vi "vision logic.vi"() -> ()   [LabVIEW 2018]
uses:
  <vilib>/Rock Robotics/Network Tables/NT Read Number.vi
  <vilib>/Rock Robotics/Network Tables/NT Read Boolean.vi
  <vilib>/Rock Robotics/Network Tables/NT Write Number.vi
  <vilib>/Rock Robotics/Network Tables/NT Write Boolean.vi
  <vilib>/Rock Robotics/WPI/Utilities/WPI_GetSetVariantRefNum.vi
  <vilib>/Rock Robotics/Network Tables/NT Write Numeric Array.vi
panel:
  out "RobotDrive Motors":dbl
  in  "Tab Control":T1(tab)
  in  "High Threshold":dbl=0.68
  in  "Low Threshold":dbl=0.63
  out "Center of Centroid":dbl
  out "Sonar1 Value":dbl
  in  "Wall (Sonar)":dbl=3.0
  in  "LX axis":dbl=0.6000000000000001 min=-1.0 max=1.0 step=0.05
  in  "LY axis":dbl=-0.45 min=-1.0 max=1.0 step=0.05
  in  "RX axis":dbl=0.45 min=-1.0 max=1.0 step=0.05
  in  "RY axis":dbl=-0.6000000000000001 min=-1.0 max=1.0 step=0.05
  in  "X axis":dbl=0.45 min=-1.0 max=1.0 step=0.05
  in  "Y axis":dbl=-0.45 min=-1.0 max=1.0 step=0.05
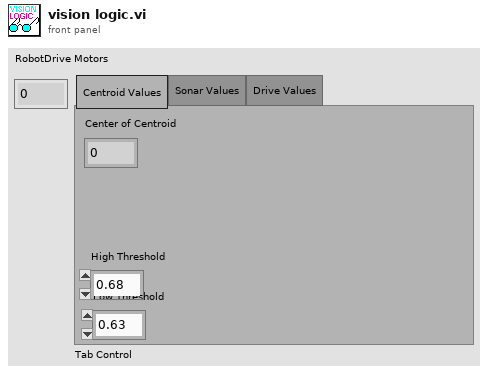
[diagram p1: front panel]
types:
  T1 = enum32{"Centroid Values", "Sonar Values", "Drive Values"}
  T2 = typedef "WPI_RobotDriveDevRef.ctl" = cluster{"DevStatus":errorcluster, "Motors[]":T3[], "Square Inputs":bool, "Max Output":dbl}
  T3 = typedef "WPI_MotorControlDeviceRef.ctl" = cluster{"DeviceStatus":errorcluster, "Type":T4, "PWM":cluster{"PWM Channel":T5, "DeadBand":T6}, "CAN":cluster{"Device Number":u8, "SetOutput VI Ref":variant, "GetOutput VI Ref":variant, "Enable VI Ref":variant, "Disable VI Ref":variant, "Data":variant}, "Invert":bool, "DIO PWM":cluster{"PWM \"Enable\" Channel":T5, "DIOChannel":T7, "PWM Rate":dbl}}
  T4 = typedef "WPI_MotorControlType.ctl" = enum16{"PWM", "CAN", "DIO PWM"}
  T5 = typedef "FPGA_DIOPWMChannel.ctl" = enum8{"PWM 0", "PWM 1", "PWM 2", "PWM 3", "PWM 4", "PWM 5", "PWM 6", "PWM 7", "PWM 8", "PWM 9", "PWM MXP 0", "PWM MXP 1", "PWM MXP 2", "PWM MXP 3", "PWM MXP 4", "PWM MXP 5", "PWM MXP 6", "PWM MXP 7", "PWM MXP 8", "PWM MXP 9", "Invalid"}
  T6 = typedef "WPI_PWMDeadband.ctl" = cluster{"Name":string, "maxPositivePwm":i32, "minPositivePwm":i32, "centerPwm":i32, "maxNegativePwm":i32, "minNegativePwm":i32, "angularRange":u16}
  T7 = typedef "FPGA_DIOChannel.ctl" = enum8{"DIO 0", "DIO 1", "DIO 2", "DIO 3", "DIO 4", "DIO 5", "DIO 6", "DIO 7", "DIO 8", "DIO 9", "DIO MXP 0", "DIO MXP 1", "DIO MXP 2", "DIO MXP 3", "DIO MXP 4", "DIO MXP 5", "DIO MXP 6", "DIO MXP 7", "DIO MXP 8", "DIO MXP 9", "DIO MXP 10", "DIO MXP 11", "DIO MXP 12", "DIO MXP 13", "DIO MXP 14", "DIO MXP 15", "SPI Port CS1", "SPI Port CS2", "SPI Port CS3", "SPI Port MISO", "SPI Port MOSI", "Invalid"}
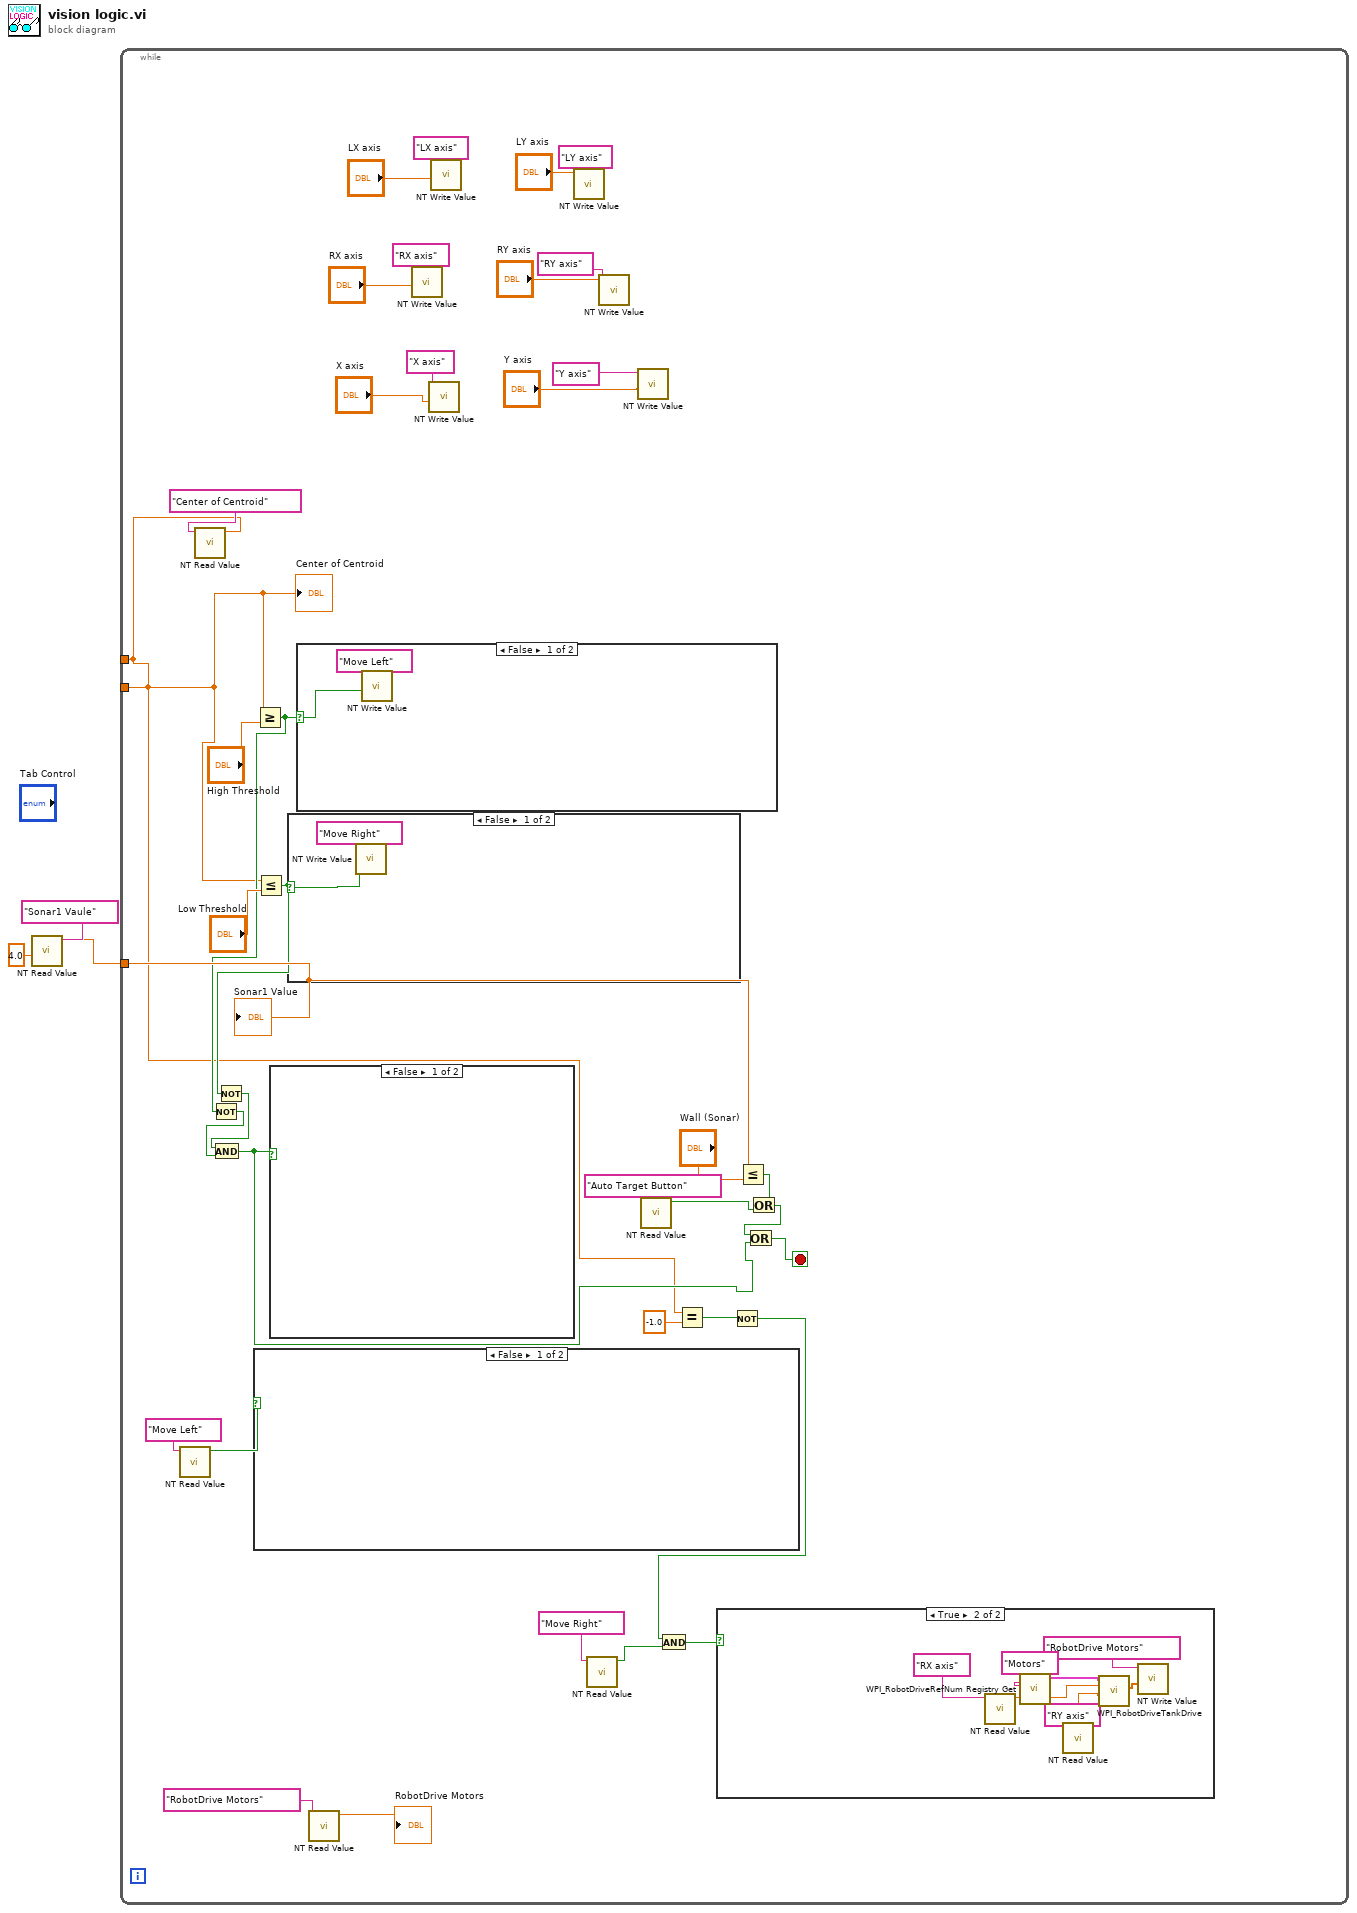
[diagram p0: block diagram]
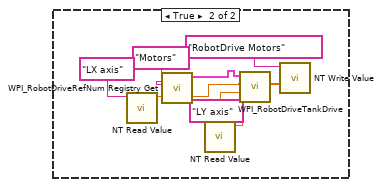
[diagram p3: hidden frame]
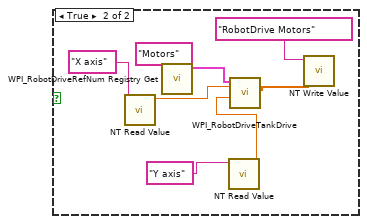
[diagram p4: hidden frame]
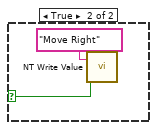
[diagram p5: hidden frame]
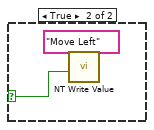
[diagram p6: hidden frame]
diagram:
  n1 = call-poly <vilib>:"NT Read Value.vi"("Default Value"=4.0, "Name"="Sonar1 Vaule") -> ("Numeric"=w2:dbl)  [unwired: 8 in, 1 out]
  n2 = while {
    tunnel: w2 -> [w36]
    tunnel: [w4] -> _
    tunnel: [w4] -> _
    stop <- w12 stop-if-true
    n3 = call-poly <vilib>:"NT Read Value.vi"("Name"="Move Left") -> ("Boolean"=w30:bool)  [unwired: 9 in, 1 out]
    n4 = call-poly <vilib>:"NT Read Value.vi"("Name"="Center of Centroid") -> ("Numeric"=w4:dbl)  [unwired: 9 in, 1 out]
    "Center of Centroid" <- w4
    n5 = case shown="False" w30 {
      frame False {
      }
      frame True {
        n6 = call-poly <vilib>:"NT Read Value.vi"("Name"="LX axis") -> ("Numeric"=w51:dbl)  [unwired: 9 in, 1 out]
        n7 = call <vilib>:"WPI_RobotDriveRefNum Registry Get.vi"("refnum name"="Motors") -> ("RobotDriveDevRef"=w52:T2)  [unwired: 1 in, 9 out]
        n8 = call-poly <vilib>:"NT Read Value.vi"("Name"="LY axis") -> ("Numeric"=w50:dbl)  [unwired: 9 in, 1 out]
        n9 = call <vilib>:"WPI_RobotDriveTankDrive.vi"("Right axis value"=w50, "Left axis value"=w51, "RobotDriveDevRef"=w52) -> ("Motor Values"=w53:dbl[])  [unwired: 6 in, 2 out]
        n10 = call-poly <vilib>:"NT Write Value.vi"("Numeric Array"=w53, "Name"="RobotDrive Motors") -> ()  [unwired: 9 in, 1 out]
      }
    }
    n11 = Greater Or Equal?(x=w4, y="High Threshold") -> (x >= y?=w32:bool)
    n12 = Not(x=w32) -> (.not. x?=w31:bool)
    n13 = Less Or Equal?(x=w4, y="Low Threshold") -> (x <= y?=w34:bool)
    n14 = Not(x=w34) -> (.not. x?=w33:bool)
    n15 = And(x=w33, y=w31) -> (x .and. y?=w10:bool)
    n16 = case shown="False" w10 {
      frame False {
      }
      frame True {
        n17 = call-poly <vilib>:"NT Read Value.vi"("Name"="X axis") -> ("Numeric"=w60:dbl)  [unwired: 9 in, 1 out]
        n18 = call <vilib>:"WPI_RobotDriveRefNum Registry Get.vi"("refnum name"="Motors") -> ("RobotDriveDevRef"=w58:T2)  [unwired: 1 in, 9 out]
        n19 = call-poly <vilib>:"NT Read Value.vi"("Name"="Y axis") -> ("Numeric"=w59:dbl)  [unwired: 9 in, 1 out]
        n20 = call <vilib>:"WPI_RobotDriveTankDrive.vi"("Right axis value"=w59, "Left axis value"=w60, "RobotDriveDevRef"=w58) -> ("Motor Values"=w61:dbl[])  [unwired: 6 in, 2 out]
        n21 = call-poly <vilib>:"NT Write Value.vi"("Numeric Array"=w61, "Name"="RobotDrive Motors") -> ()  [unwired: 9 in, 1 out]
      }
    }
    n22 = case shown="False" w34 {
      selector: w34 -> [w66 w69]
      frame False {
        n23 = call-poly <vilib>:"NT Write Value.vi"("Boolean"=w66, "Name"="Move Right") -> ()  [unwired: 9 in, 1 out]
      }
      frame True {
        n24 = call-poly <vilib>:"NT Write Value.vi"("Boolean"=w69, "Name"="Move Right") -> ()  [unwired: 9 in, 1 out]
      }
    }
    n25 = case shown="False" w32 {
      selector: w32 -> [w70 w73]
      frame False {
        n26 = call-poly <vilib>:"NT Write Value.vi"("Boolean"=w70, "Name"="Move Left") -> ()  [unwired: 9 in, 1 out]
      }
      frame True {
        n27 = call-poly <vilib>:"NT Write Value.vi"("Boolean"=w73, "Name"="Move Left") -> ()  [unwired: 9 in, 1 out]
      }
    }
    n28 = call-poly <vilib>:"NT Read Value.vi"("Name"="RobotDrive Motors") -> ("Numeric"=→"RobotDrive Motors":dbl)  [unwired: 9 in, 1 out]
    n29 = call-poly <vilib>:"NT Write Value.vi"("Numeric"="RX axis", "Name"="RX axis") -> ()  [unwired: 9 in, 1 out]
    n30 = call-poly <vilib>:"NT Write Value.vi"("Numeric"="X axis", "Name"="X axis") -> ()  [unwired: 9 in, 1 out]
    n31 = call-poly <vilib>:"NT Write Value.vi"("Numeric"="LX axis", "Name"="LX axis") -> ()  [unwired: 9 in, 1 out]
    n32 = call-poly <vilib>:"NT Write Value.vi"("Numeric"="LY axis", "Name"="LY axis") -> ()  [unwired: 9 in, 1 out]
    n33 = call-poly <vilib>:"NT Read Value.vi"("Name"="Move Right") -> ("Boolean"=w8:bool)  [unwired: 9 in, 1 out]
    n34 = call-poly <vilib>:"NT Write Value.vi"("Numeric"="RY axis", "Name"="RY axis") -> ()  [unwired: 9 in, 1 out]
    n35 = call-poly <vilib>:"NT Write Value.vi"("Numeric"="Y axis", "Name"="Y axis") -> ()  [unwired: 9 in, 1 out]
    n36 = call-poly <vilib>:"NT Read Value.vi"("Name"="Auto Target Button") -> ("Boolean"=w41:bool)  [unwired: 9 in, 1 out]
    n37 = Equal?(x=w4, y=-1.0) -> (x = y?=w7:bool)
    n38 = Not(x=w7) -> (.not. x?=w6:bool)
    n39 = And(x=w6, y=w8) -> (x .and. y?=w9:bool)
    n40 = case shown="True" w9 {
      frame False {
      }
      frame True {
        n41 = call-poly <vilib>:"NT Read Value.vi"("Name"="RX axis") -> ("Numeric"=w43:dbl)  [unwired: 9 in, 1 out]
        n42 = call <vilib>:"WPI_RobotDriveRefNum Registry Get.vi"("refnum name"="Motors") -> ("RobotDriveDevRef"=w44:T2)  [unwired: 1 in, 9 out]
        n43 = call-poly <vilib>:"NT Read Value.vi"("Name"="RY axis") -> ("Numeric"=w42:dbl)  [unwired: 9 in, 1 out]
        n44 = call <vilib>:"WPI_RobotDriveTankDrive.vi"("Right axis value"=w42, "Left axis value"=w43, "RobotDriveDevRef"=w44) -> ("Motor Values"=w45:dbl[])  [unwired: 6 in, 2 out]
        n45 = call-poly <vilib>:"NT Write Value.vi"("Numeric Array"=w45, "Name"="RobotDrive Motors") -> ()  [unwired: 9 in, 1 out]
      }
    }
    n46 = Less Or Equal?(x=w36, y="Wall (Sonar)") -> (x <= y?=w39:bool)
    n47 = Or(x=w39, y=w41) -> (x .or. y?=w13:bool)
    n48 = Or(x=w13, y=w10) -> (x .or. y?=w12:bool)
    "Sonar1 Value" <- w36
  }
